vi "CannonProjectileGame.vi"() -> ()   [LabVIEW 2018]
panel:
  out "Distance":dbl
  out "?":cluster{dbl[], dbl[]}(graph)
  out "Score":dbl
  out "Attempt":i32
  out "Wind (mph)":dbl
  out "Target Distance (m)":dbl
  in  "?":bool
  in  "?":bool
  in  "Height (m)":dbl
  in  "Power":dbl
  in  "Angle (deg)":dbl
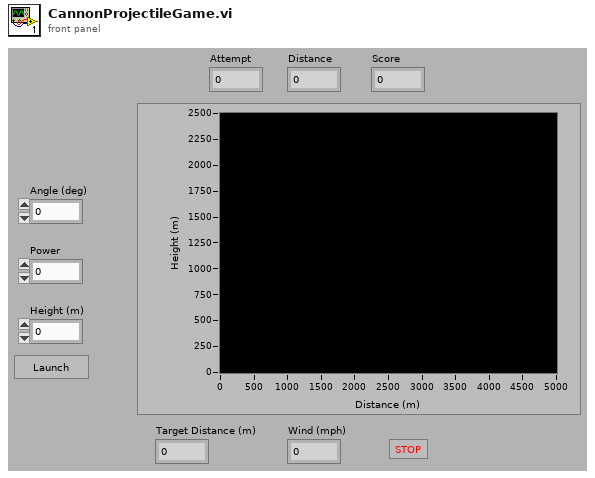
[diagram p1: front panel]
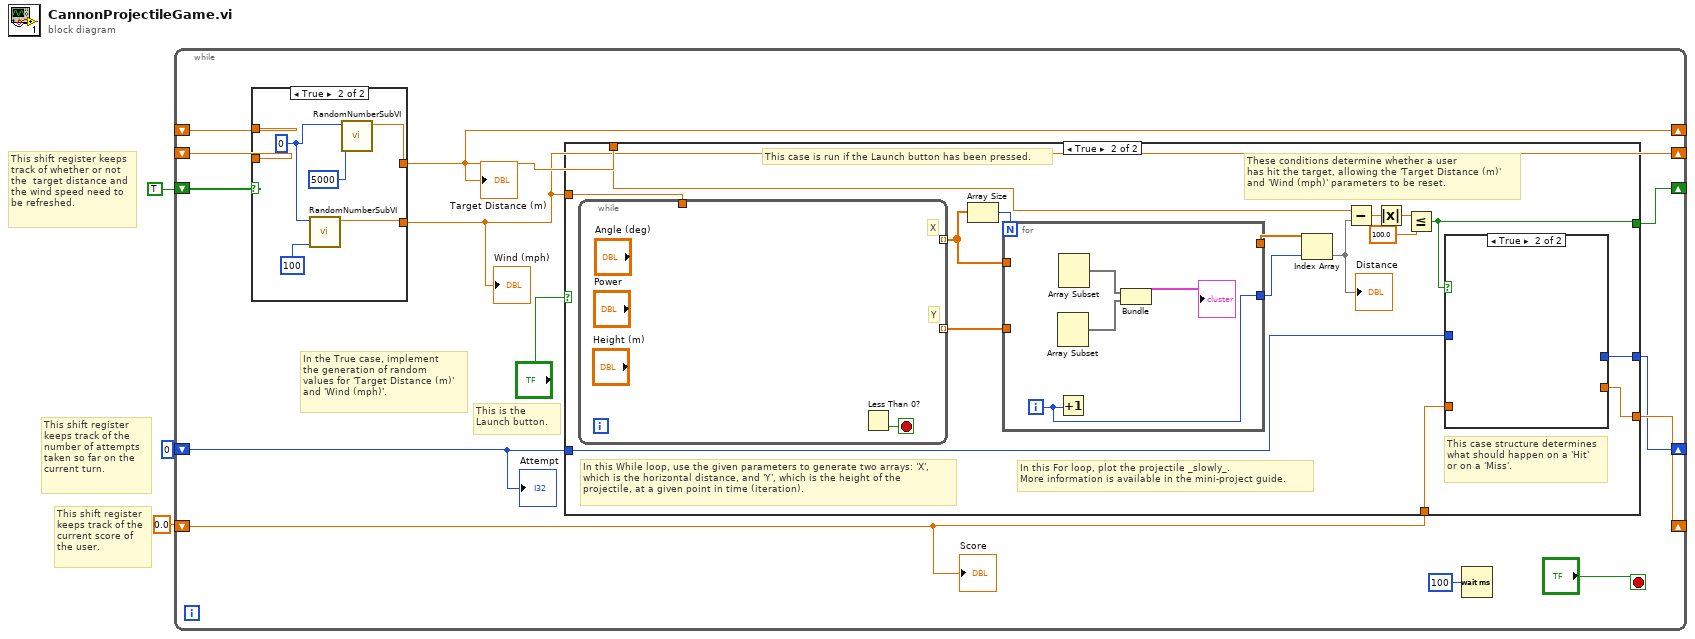
[diagram p0: block diagram]
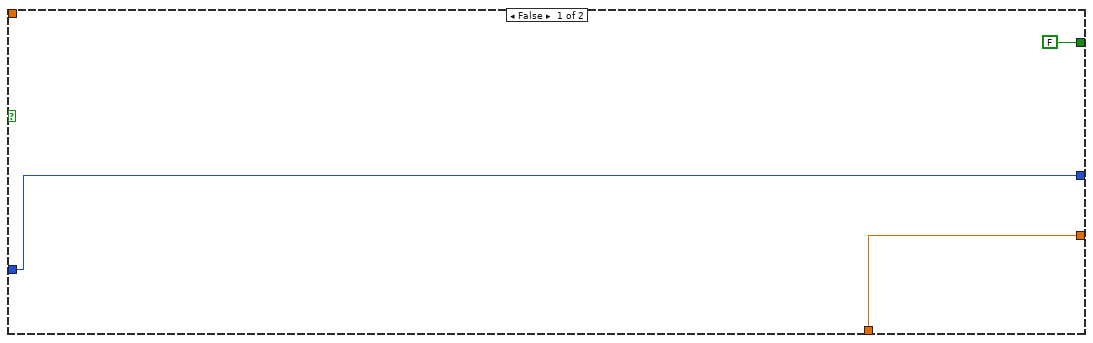
[diagram p3: hidden frame]
diagram:
  # "This shift register keeps\ntrack of whether or not\nthe  target distance and\nthe wind speed need to\nbe refreshed."
  # "This shift register\nkeeps track of the\ncurrent score of\nthe user."
  # "This shift register\nkeeps track of the\nnumber of attempts\ntaken so far on the\ncurrent turn."
  n1 = while {
    shift-right: [w14] -> _
    shift-left: 0.0 -> [w13]
    shift-right: [w12] -> _
    shift-left: 0 -> [w11]
    shift-right: [w9] -> _
    shift-left: TRUE -> [w4]
    shift-right: [w6] -> _
    shift-left: _ -> [w8]
    shift-right: [w5] -> _
    shift-left: _ -> [w7]
    stop <- "?" stop-if-true
    # "This is the Launch button."
    # "In the True case, implement\nthe generation of random\nvalues for 'Target Distance (m)'\nand 'Wind (mph)'."
    n2 = case shown="True" w4 {
      tunnel: [w18 w22] -> w6
      tunnel: [w17 w23] -> w5
      tunnel: w8 -> [w18 _]
      tunnel: w7 -> [w17 _]
      frame False {
      }
      frame True {
        w21 = 0
        n3 = call "RandomNumberSubVI.vi"("Maximum"=100, "Minimum"=w21) -> ("Random Number"=w23:dbl)  [unwired: 9 in]
        n4 = call "RandomNumberSubVI.vi"("Maximum"=5000, "Minimum"=w21) -> ("Random Number"=w22:dbl)  [unwired: 9 in]
      }
    }
    "Target Distance (m)" <- w6
    "Wind (mph)" <- w5
    n5 = case shown="True" "?" {
      tunnel: w6 -> [_ w41]
      tunnel: w5 -> [_ w42]
      tunnel: [w26 w37] -> w12
      tunnel: w11 -> [w26 w28]
      tunnel: [w25 w30] -> w14
      tunnel: w13 -> [w25 w29]
      tunnel: [FALSE w27] -> w9
      frame False {
      }
      frame True {
        # "These conditions determine whether a user\nhas hit the target, allowing the 'Target Distance (m)'\nand 'Wind (mph)' parameters to be reset."
        # "This case is run if the Launch button has been pressed."
        # "This case structure determines\nwhat should happen on a 'Hit'\nor on a 'Miss'."
        # "In this For loop, plot the projectile _slowly_.\nMore information is available in the mini-project guide."
        # "In this While loop, use the given parameters to generate two arrays: 'X',\nwhich is the horizontal distance, and 'Y', which is the height of the\nprojectile, at a given point in time (iteration)."
        n6 = while {
          tunnel: w42 -> [_]
          tunnel: [_] -> w31 mode=indexing
          tunnel: [_] -> w36 mode=indexing
          stop <- w47 stop-if-true
          # "Y"
          # "X"
          n7 = Less Than 0?() -> (x < 0?=w47:bool)  [unwired: 1 in]
        }
        n8 = Array Size(array=w31) -> (size(s)=w32:i32)
        n9 = for {
          N: w32 -> [_]
          tunnel: w31 -> [_]
          tunnel: w36 -> [_]
          tunnel: [_] -> w35
          tunnel: [w44] -> w34
          i -> [w44]
          n10 = Array Subset() -> (w45:void[])  [unwired: 3 in]
          n11 = Increment(x=w44) -> ()  [unwired: 1 out]
          n12 = Array Subset() -> (w46:void[])  [unwired: 3 in]
          n13 = Bundle(w46, w45) -> (→"?":cluster{void[], void[]})  [unwired: 1 out]
        }
        n14 = Index Array(array=w35, index=w34) -> (element=w33)
        "Distance" <- w33
        n15 = Subtract(x=w41, y=w33) -> (x-y=w40:dbl)
        n16 = Absolute Value(x=w40) -> (abs(x)=w39:dbl)
        n17 = Less Or Equal?(x=w39, y=100.0) -> (x <= y?=w27:bool)
        n18 = case shown="True" w27 {
          tunnel: [_ _] -> w37
          tunnel: w28 -> [_ _]
          tunnel: [_ _] -> w30
          tunnel: w29 -> [_ _]
          frame False {
          }
          frame True {
          }
        }
      }
    }
    n19 = Wait (ms)(milliseconds to wait=u32 100) -> ()  [unwired: 1 out]
    "Score" <- w13
    "Attempt" <- w11
  }
